vi "Tektronix DPO MSO 2000 4000 Series Transfer Current Waveform Example dave.vi"() -> ()   [LabVIEW 2011]
doc: "This example illustrates how to transfer the current waveform on an oscilloscope using the following steps:\n\n1. Specify a valid VISA session. \n2. Specify a channel. \n3. Specify a time-out value for reading waveform.\n4. Run the VI. The graph displays the waveform you acquire."
uses:
  <instrlib>/Tektronix DPO MSO 2000 4000 Series/Public/Data/Data_Low Level/Fetch Waveform (Waveform Data Type).vi
  <instrlib>/Tektronix DPO MSO 2000 4000 Series/Tektronix DPO MSO 2000 4000 Series.lvlib
panel:
  in  "Channel (0: Channel 1)":u16(ring) items=["Channel 1", "Channel 2", "Channel 3", "Channel 4", "Math", "Reference 1", "Reference 2", "Reference 3", "Reference 4", "D0", "D1", "D2", "D3", "D4", "D5", "D6", "D7", "D8", "D9", "D10", "D11", "D12", "D13", "D14", "D15", "Amplitude", "Frequency", "Phase", "Normal", "Average", "Maximum Peak Hold", "Minimum Peak Hold"]
  in  "Maximum Time (10000ms)":u32=10000
  in  "VISA Resource Name":refnum<visa-resource-name>
  out "Waveform Graph":waveform(dbl)(graph)
  # "(c) 2006 - 2012. National Instruments Corporation. ALL RIGHTS RESERVED."
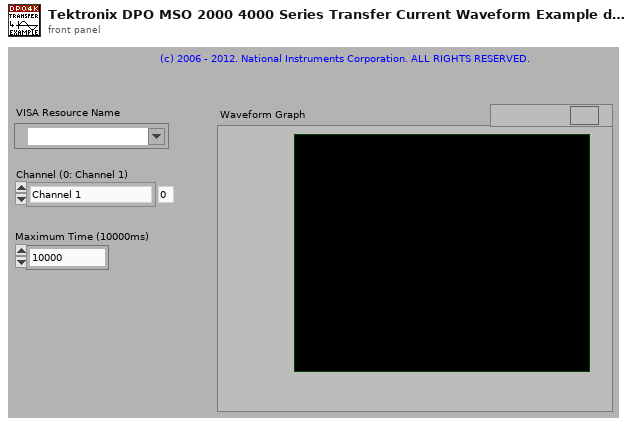
[diagram p1: front panel]
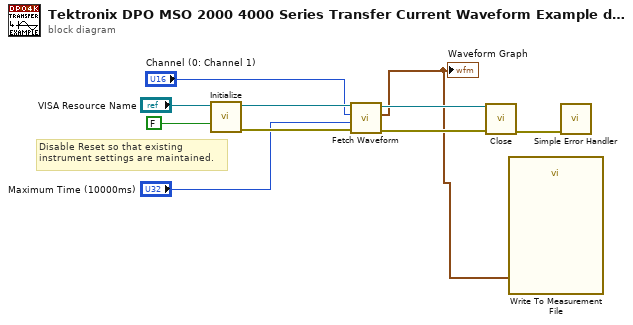
[diagram p0: block diagram]
diagram:
  # "Disable Reset so that existing\ninstrument settings are maintained."
  n1 = call <instrlib>:"Initialize.vi"("Reset (True)"=FALSE ("Reset? (T: Yes)"), "VISA resource name"="VISA Resource Name") -> ("error out"=w6:errorcluster, "VISA resource name out"=w7:refnum<visa-resource-name>)  [unwired: 8 in]
  n2 = call-poly <instrlib>:"Fetch Waveform.vi"("error in (no error)"=w6, "Maximum Time (10000ms)"="Maximum Time (10000ms)", "Channel (0: Channel 1)"="Channel (0: Channel 1)", "VISA resource name"=w7) -> ("error out"=w5:errorcluster, "Waveform Data"=w1:waveform(dbl), "VISA resource name out"=w2:refnum<visa-resource-name>)  [unwired: 5 in]
  "Waveform Graph" <- w1
  n3 = call <instrlib>:"Close.vi"("error in (no error)"=w5, "VISA resource name"=w2) -> ("error out"=w9:errorcluster)  [unwired: 9 in]
  n4 = call "Write To Measurement File"("Signals"=w1) -> ()  [unwired: 16 in, 3 out]
  n5 = call <vilib>:"Simple Error Handler.vi"("error in (no error)"=w9) -> ()  [unwired: 4 in, 5 out]
